vi "Set_Tunnel_Speed.vi"(3 "Mode":T1, 5 "Tunnel Velocity m/s":dbl min=0.0 max=50.0 format="%.2f") -> (0 "Error String":string)   [LabVIEW 2010]
doc: "This is an example of using features of the VI Server as a client. It shows how you might browse from one or more applications that may be exporting data from one or more data stations. \n\nThe example shows how to query a server for its list of exported VIs, how to get references to the VIs, and how call them with the Call By Reference function."
uses:
  Sub VIs/ADAM Controls/Tunnel_speed_mode.ctl
  Anemometry/Anemometry Sub Vis/File/Setup_Filetype.ctl
  Sub VIs/ADAM Controls/Channel_State.ctl
  Sub VIs/ADAM Controls/Calib_type_ADAM.ctl
  Sub VIs/ADAM Controls/Module_type_ADAM.ctl
  Sub VIs/ADAM Controls/Ch_description_ADAM.ctl
  Sub VIs/ADAM Controls/Function_ADAM.ctl
  Sub VIs/ADAM Controls/Address.ctl
  Anemometry/Anemometry Sub Vis/Controls/Global_mode.ctl
  Sub VIs/ADAM Controls/Update_scan_value.ctl
  Anemometry/Anemometry Sub Vis/Globals/Preference_global.vi
  Anemometry/Anemometry Sub Vis/Globals/Trav_pos_global.vi
  Anemometry/Anemometry Sub Vis/Globals/Constants_global.vi
  <vilib>/Analysis/NI_AALBase.lvlib
panel:
  in  "Set EnFlo Tun Speed":refnum<vi>
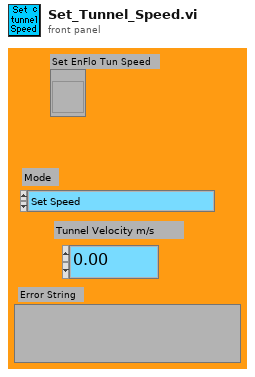
[diagram p1: front panel]
types:
  T1 = typedef "Tunnel_speed_mode.ctl" = enum16{"Set Speed", "Set Speed then wait", "Is tunnel speed allowable?"}
  T2 = typedef "Setup_Filetype.ctl" = enum16{"Measurement Setups", "Calibration Setups", "General", "Results File Plotter Setups", "Speed Calib Tweaks"}
  T3 = typedef "Channel_State.ctl" = enum16{"On", "Off", "Always On", "Always Off"}
  T4 = typedef "Calib_type_ADAM.ctl" = enum16{"Raw", "Bx + A", "Cx^2 + Bx + A", "Dx^3 + Cx^2 + Bx + A", "In Band", "Hi-Tec Q", "Hi-Tec M_dot", "Text"}
  T5 = typedef "Module_type_ADAM.ctl" = enum16{"4011", "4012", "4013", "4014", "4016", "4017", "4018", "4021", "4050", "4052", "4053", "4060", "4080", "5000", "5017", "5018", "5024", "5051", "5056", "5060", "6060", "Tracker", "WEST", "GILL", "JEM", "VICI", "Vaisala", "DRUCK", "Run VI Named:", "IR2100", "PPT", "Comparator", "VIRTUAL", "Hold Value", "Read A", "Read Ch", "Coded", "Client Info", "Web Client", "X10", "Test"}
  T6 = typedef "Ch_description_ADAM.ctl" = cluster{"Ch Name":string, "Type":T5, "Function":T7, "Ch State":T3, "Calibration type":T4, "A":dbl, "B":dbl, "C":dbl, "D":dbl, "Comments":string, "Address":T8, "String":string, "Duty":u16}
  T7 = typedef "Function_ADAM.ctl" = enum16{"Analogue Input", "Digital Input", "Event counter", "Event rate", "Analogue Output", "Digital Output", "Relay Output"}
  T8 = typedef "Address.ctl" = cluster{"Main":i32, "Ch.":i32, "Sub":i32, "Port Name":string}
  T9 = typedef "Global_mode.ctl" = enum16{"Read Global", "Load Global From File", "Write Global to File"}
  T10 = typedef "Update_scan_value.ctl" = cluster{"Channel Name":string, "New Value":dbl}
  T11 = typedef "Server_Comms.ctl" = enum16{"Server Link Healthy", "Do Not Link To Server"}
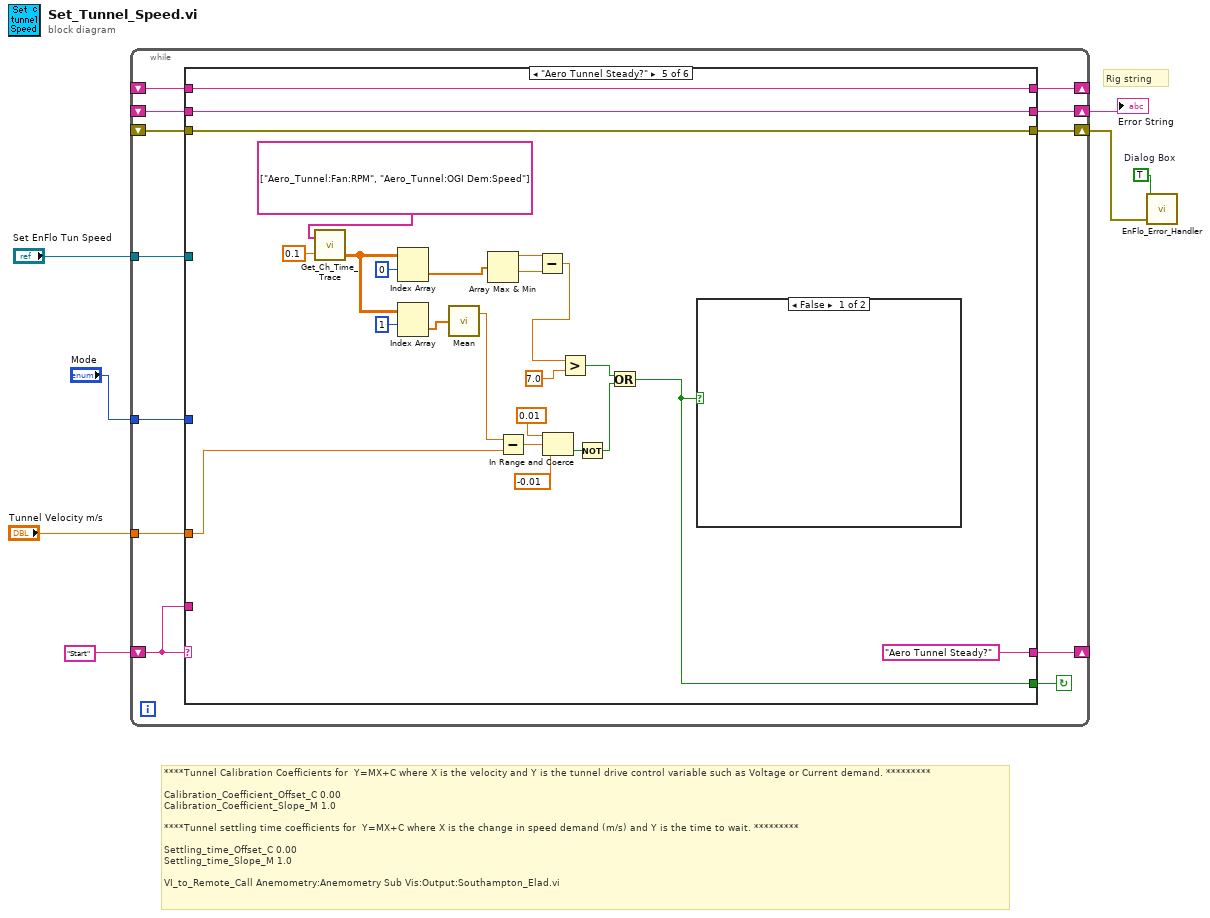
[diagram p0: block diagram]
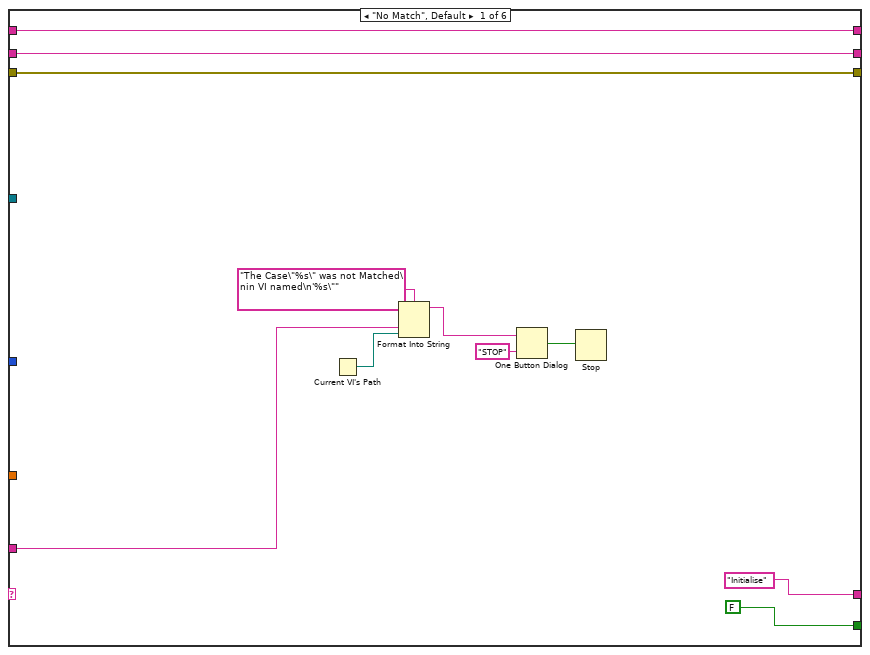
[diagram p2: hidden frame]
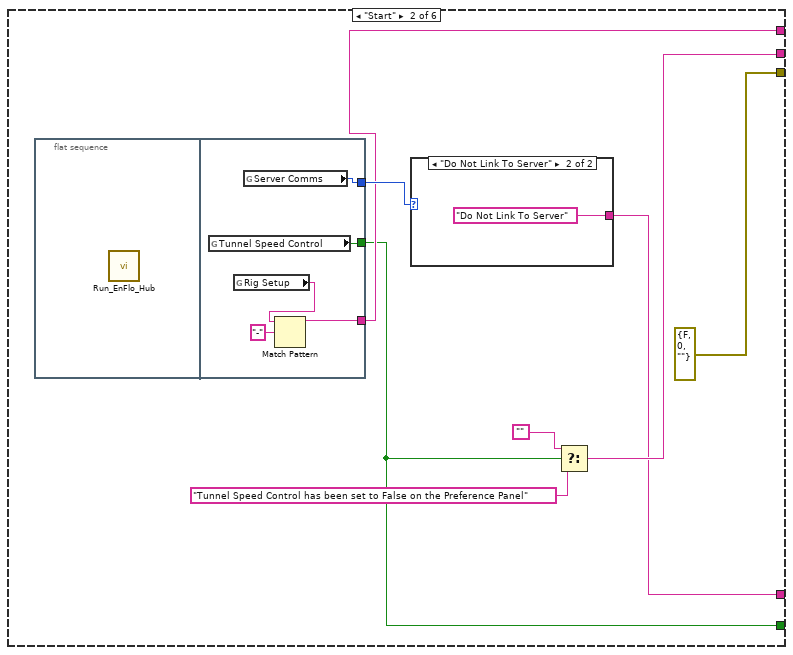
[diagram p3: hidden frame]
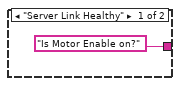
[diagram p4: hidden frame]
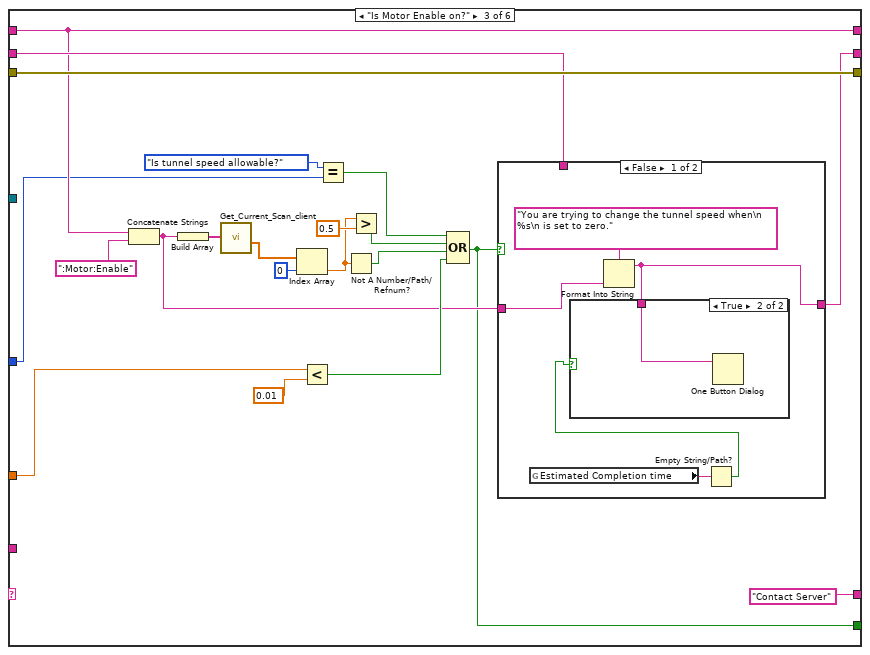
[diagram p5: hidden frame]
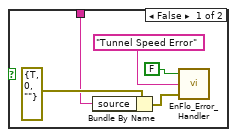
[diagram p6: hidden frame]
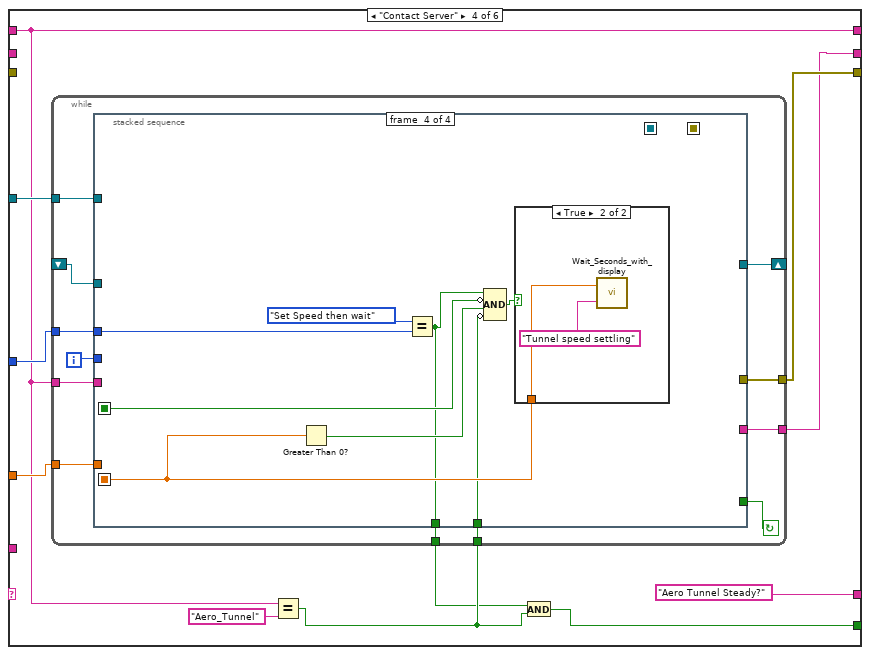
[diagram p8: hidden frame]
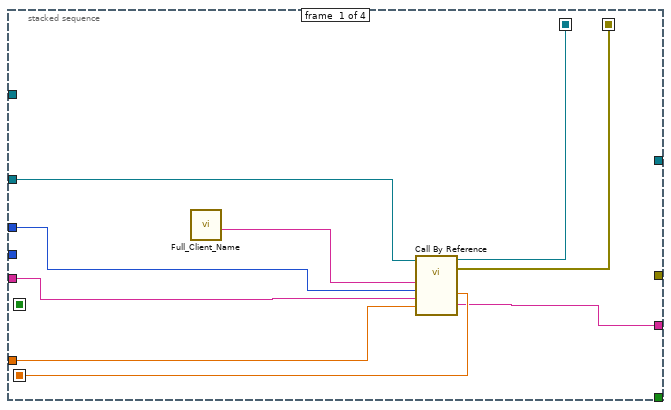
[diagram p9: hidden frame]
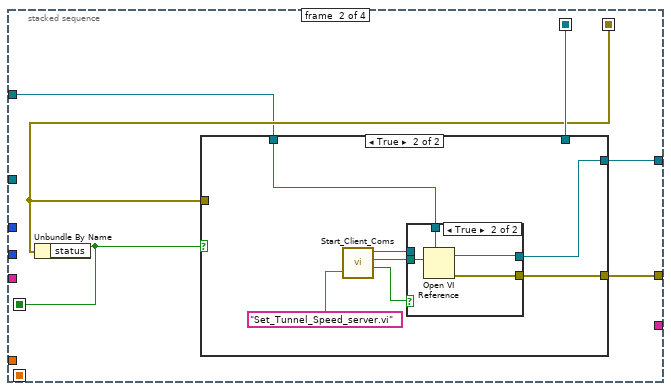
[diagram p10: hidden frame]
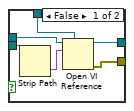
[diagram p12: hidden frame]
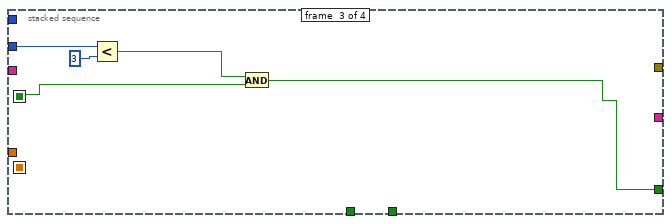
[diagram p13: hidden frame]
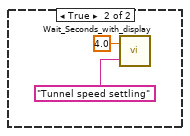
[diagram p15: hidden frame]
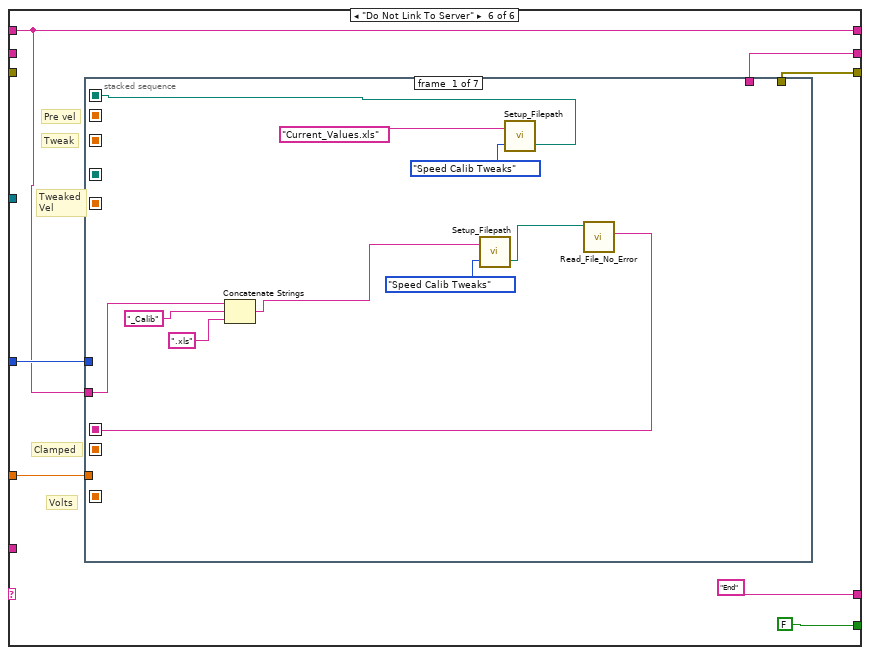
[diagram p16: hidden frame]
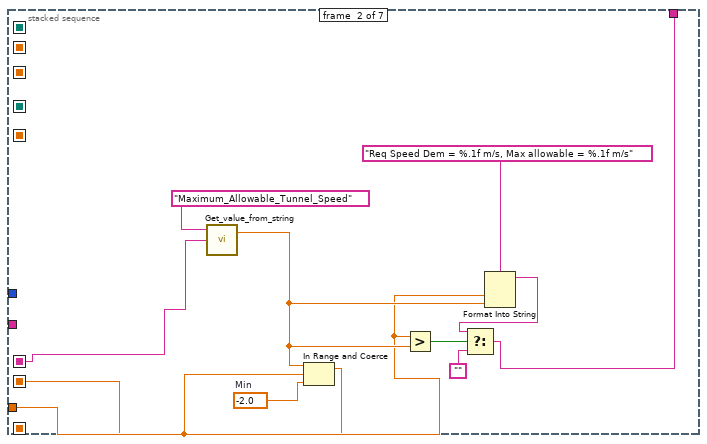
[diagram p17: hidden frame]
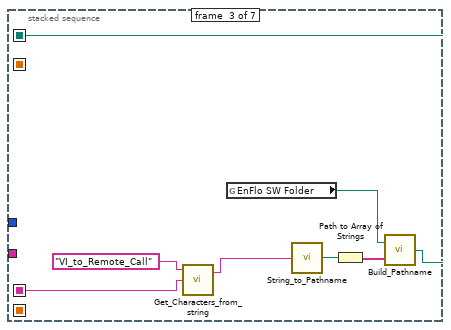
[diagram p18: hidden frame]
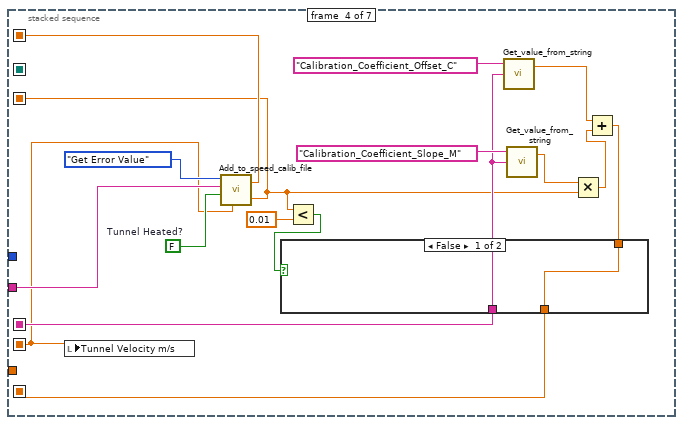
[diagram p19: hidden frame]
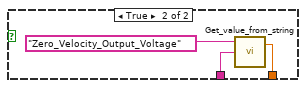
[diagram p20: hidden frame]
diagram:
  w7 = TRUE  # Dialog Box
  # "Rig string"
  # "****Tunnel Calibration Coefficients for  Y=MX+C where X is the velocity and Y is the tunnel drive control variable such as Voltage or Current demand. *********\n\nCalibration_Coefficient_Offset_C\t0.00\nCalibration_Coefficient_Slope_M\t1.0\n\n****Tunnel settling time coefficients for  Y=MX+C where X is the change in speed demand (m/s) and Y is the time to wait. *********\n\nSettling_time_Offset_C\t0.00\nSettling_time_Slope_M\t1.0\n\nVI_to_Remote_Call\tAnemometry:Anemometry Sub Vis:Output:Southampton_Elad.vi"
  n1 = while {
    shift-left: "Start" -> [w18]
    shift-right: [w19] -> _
    shift-right: [w17] -> w5
    shift-left: _ -> [w16]
    shift-right: [w15] -> w4
    shift-left: _ -> [w10]
    tunnel: "Mode" -> [w14]
    tunnel: "Tunnel Velocity m/s" -> [w13]
    shift-right: [w12] -> _
    shift-left: _ -> [w11]
    tunnel: "Set EnFlo Tun Speed" -> [w8]
    stop <- w9 continue-if-true
    n2 = case shown="\"Aero Tunnel Steady?\"" w18 {
      tunnel: [FALSE w35 w51 w79 w156 FALSE] -> w9
      tunnel: ["Initialise" w31 "Contact Server" ("f") "Aero Tunnel Steady?" ("f") "Aero Tunnel Steady?" ("f") "End"] -> w19
      tunnel: w18 -> [w25 _ _ _ _ _]
      tunnel: [w22 w33 w53 w86 w172 w179] -> w17
      tunnel: w16 -> [w22 _ w52 _ w172 _]
      tunnel: [w20 errorcluster {"status"=FALSE, "code"=0, "source"=""} ("error out") w55 w87 w171 w178] -> w15
      tunnel: w14 -> [_ _ w48 w89 _ w181]
      tunnel: w13 -> [_ _ w56 w88 w163 w180]
      tunnel: [w21 w36 w50 w83 w173 w177] -> w12
      tunnel: w11 -> [w21 _ w50 w83 w173 w177]
      tunnel: w10 -> [w20 _ w55 _ w171 _]
      tunnel: w8 -> [_ _ _ w85 _ _]
      frame "No Match", Default {
        n3 = Current VI's Path() -> (path=w24:path)
        n4 = Format Into String(format string="The Case\"%s\" was not Matched\nin VI named\n'%s\"" ("Format String"), w25, w24) -> (resulting string=w28:string)  [unwired: 2 in, 1 out]
        n5 = One Button Dialog(message=w28, button name ("OK")="STOP") -> (true=w26:bool)
        n6 = Stop(stop? (T)=w26) -> ()
      }
      frame "Start" {
        n7 = flat-sequence {
          tunnel: [w45] -> w38
          tunnel: [w44] -> w35
          tunnel: [w41] -> w36
          frame #0 {
            n8 = call "Run_EnFlo_Hub.vi"() -> ()  [unwired: 8 out]
          }
          frame #1 {
            n9 = global read "Preference_global.vi" "Tunnel Speed Control"() -> (w44:bool)
            n10 = global read "Preference_global.vi" "Rig Setup"() -> (w43:string)
            n11 = global read "Preference_global.vi" "Server Comms"() -> (w45:T11)
            n12 = Match Pattern(string=w43, regular expression="-") -> (before substring=w41:string)  [unwired: 4 out]
          }
        }
        n13 = case shown="\"Do Not Link To Server\"" w38 {
          tunnel: ["Is Motor Enable on?" "Do Not Link To Server"] -> w31
          frame "Server Link Healthy" {
          }
          frame "Do Not Link To Server" {
          }
        }
        n14 = Select(t="", s=w35, f="Tunnel Speed Control has been set to False on the Preference Panel" ("Error String")) -> (s? t:f=w33:string)
      }
      frame "Is Motor Enable on?" {
        n15 = Concatenate Strings(w50, ":Motor:Enable" ("string")) -> (w54:string)
        n16 = Build Array(w54) -> (w58:string[])
        n17 = call "Get_Current_Scan_client.vi"("ADAM Ch Names"=w58) -> ("Numerical Values"=w59:dbl[])  [unwired: 3 out]
        n18 = Index Array(array=w59, index=0) -> (element=w61:dbl)
        n19 = Less?(x=w56, y=0.01) -> (x < y?=w66:bool)
        n20 = Equal?(x=Tunnel_speed_mode."Is tunnel speed allowable?" ("Mode"), y=w48) -> (x = y?=w47:bool)
        n21 = Not A Number/Path/Refnum?(number/path/refnum=w61) -> (NaN/Path/Refnum?=w63:bool)
        n22 = Greater?(x=w61, y=0.5) -> (0:w64:bool)
        n23 = Compound Arithmetic op=OR(w47, w64, w63, w66) -> (w51:bool)
        n24 = case shown="False" w51 {
          tunnel: w54 -> [w70 _]
          tunnel: [w67 w78] -> w53
          tunnel: w52 -> [_ w78]
          frame False {
            n25 = global read "Trav_pos_global.vi" "Estimated Completion time"() -> (w69:string)
            n26 = Format Into String(format string="You are trying to change the tunnel speed when\n %s\n is set to zero.", w70) -> (resulting string=w67:string)  [unwired: 2 in, 1 out]
            n27 = Empty String/Path?(string/path=w69) -> (empty?=w68:bool)
            n28 = case shown="True" w68 {
              tunnel: w67 -> [w73 w77]
              frame False {
                n29 = Bundle By Name(cluster=errorcluster {"status"=TRUE, "code"=0, "source"=""} ("error in (no error)"), "source"=w73) -> (w74:errorcluster)
                n30 = call "EnFlo_Error_Handler.vi"("error in (no error)"=w74, "Error Type"="Tunnel Speed Error", "Dialog Box (T)"=FALSE) -> ()  [unwired: 3 out]
              }
              frame True {
                n31 = One Button Dialog(message=w77) -> ()  [unwired: 2 out]
              }
            }
          }
          frame True {
          }
        }
      }
      frame "Contact Server" {
        n32 = Equal?(x=w83, y="Aero_Tunnel") -> (x = y?=w81:bool)
        n33 = while {
          tunnel: w89 -> [w96]
          tunnel: w88 -> [w97]
          tunnel: [w98] -> w87
          shift-left: _ -> [w93]
          shift-right: [w101] -> _
          tunnel: [w95] -> w86
          tunnel: w83 -> [w94]
          tunnel: w85 -> [w92]
          tunnel: w81 -> [w91]
          tunnel: [w90] -> w80
          i -> [w100]
          stop <- w99 continue-if-true
          n34 = stacked-sequence {
            seq-local: [w109 _ _ _] -> [_ w115 _ _]
            seq-local: [w108 _ _ _] -> [_ w113 _ _]
            seq-local: [_ w114 _ _] -> [_ _ w137 w144]
            seq-local: [w105 _ _ _] -> [_ _ _ w147]
            tunnel: w93 -> [w110 _ _ _]
            tunnel: [_ w116 _ _] -> w101
            tunnel: w100 -> [_ _ w138 _]
            tunnel: [_ _ w136 _] -> w99
            tunnel: [_ w112 _ _] -> w98
            tunnel: w97 -> [w106 _ _ _]
            tunnel: w96 -> [w102 _ _ w148]
            tunnel: [w104 _ _ _] -> w95
            tunnel: w94 -> [w103 _ _ _]
            tunnel: w92 -> [_ w111 _ _]
            tunnel: w91 -> [_ _ _ w142]
            tunnel: [_ _ _ w141] -> w90
            frame #0 {
              n35 = call "Full_Client_Name.vi"() -> ("Client Name"=w107:string)
              n36 = call-by-ref "?"(reference=w110, "Tunnel Velocity m/s"=w106, "Rig Name"=w103, "Mode"=w102, "Client Name"=w107) -> (reference out=w109:refnum<vi>, error out=w108:errorcluster, "Error String"=w104:string, "Settling Time (s)"=w105:dbl)  [unwired: 1 in, 1 out]
            }
            frame #1 {
              n37 = Unbundle By Name(w113) -> ("status"=w114:bool)
              n38 = case shown="True" w114 {
                tunnel: [w117 w121] -> w116
                tunnel: w115 -> [w117 _]
                tunnel: [w118 w120] -> w112
                tunnel: w113 -> [w118 _]
                tunnel: w111 -> [_ w119]
                frame False {
                }
                frame True {
                  n39 = call "Start_Client_Coms.vi"("VI name to run on server"="Set_Tunnel_Speed_server.vi") -> ("LabVIEW application reference"=w123:refnum<vi>, "Checked VI name"=w124:path, "Local Call"=w122:bool)  [unwired: 1 in, 1 out]
                  n40 = case shown="True" w122 {
                    tunnel: [w130 w135] -> w121
                    tunnel: w119 -> [w128 w134]
                    tunnel: w124 -> [w127 w133]
                    tunnel: w123 -> [w126 _]
                    tunnel: [w129 w132] -> w120
                    frame False {
                      n41 = Strip Path(path=w127) -> (name=w131:string)  [unwired: 1 out]
                      n42 = Open VI Reference(type specifier VI Refnum (for type only)=w128, application reference (local)=w126, vi path=w131) -> (vi reference=w130:refnum<vi>, error out=w129:errorcluster)  [unwired: 1 in, 2 out]
                    }
                    frame True {
                      n43 = Open VI Reference(type specifier VI Refnum (for type only)=w134, vi path=w133) -> (vi reference=w135:refnum<vi>, error out=w132:errorcluster)  [unwired: 1 in, 3 out]
                    }
                  }
                }
              }
            }
            frame #2 {
              n44 = Less?(x=w138, y=3) -> (x < y?=w140:bool)
              n45 = And(x=w140, y=w137) -> (x .and. y?=w136:bool)
            }
            frame #3 {
              n46 = Greater Than 0?(x=w147) -> (x > 0?=w143:bool)
              n47 = Equal?(x=Tunnel_speed_mode."Set Speed then wait" ("Mode"), y=w148) -> (x = y?=w141:bool)
              n48 = Compound Arithmetic op=AND(w141, invert w144, w143, invert w142) -> (w145:bool)
              n49 = case shown="True" w145 {
                tunnel: w147 -> [_ w149]
                frame False {
                }
                frame True {
                  n50 = call "Wait_Seconds_with_display.vi"("Message"="Tunnel speed settling", "Seconds to wait"=w149) -> ()  [unwired: 2 out]
                }
              }
            }
          }
        }
        n51 = And(x=w80, y=w81) -> (x .and. y?=w79:bool)
      }
      frame "Aero Tunnel Steady?" {
        n52 = call "Get_Ch_Time_Trace.vi"("Desired Ch Names"=string[] ["Aero_Tunnel:Fan:RPM", "Aero_Tunnel:OGI Dem:Speed"] ("ADAM Ch Names"), "History Length (mins)"=0.1) -> ("Output array"=w166:dbl[][])  [unwired: 2 out]
        n53 = Index Array(array=w166, index (row)=0) -> (element=w162:dbl[])  [unwired: 1 in]
        n54 = Index Array(array=w166, index (row)=1) -> (element=w165:dbl[])  [unwired: 1 in]
        n55 = call <vilib>:"Mean.vi"("X"=w165) -> ("mean"=w164:dbl)  [unwired: 1 out]
        n56 = Array Max & Min(array=w162) -> (max value=w161:dbl, min value=w160:dbl)  [unwired: 2 out]
        n57 = Subtract(x=w164, y=w163) -> (x-y=w153:dbl)
        n58 = Subtract(x=w161, y=w160) -> (x-y=w159:dbl)
        n59 = In Range and Coerce(upper limit=0.01, x=w153, lower limit=-0.01) -> (In Range?=w152:bool)  [unwired: 1 out]
        n60 = Greater?(x=w159, y=7.0) -> (0:w157:bool)
        n61 = Not(x=w152) -> (.not. x?=w151:bool)
        n62 = Or(x=w157, y=w151) -> (x .or. y?=w156:bool)
        n63 = case shown="False" w156 {
          frame False {
          }
          frame True {
            n64 = call "Wait_Seconds_with_display.vi"("Message"="Tunnel speed settling", "Seconds to wait"=4.0) -> ()  [unwired: 2 out]
          }
        }
      }
      frame "Do Not Link To Server" {
        # "Clamped"
        # "Pre vel"
        # "Tweak"
        # "Tweaked\nVel"
        # "Volts"
        n65 = stacked-sequence {
          seq-local: [w190 _ _ _ _ _ _] -> [_ w204 w210 w218 w234 w293 _]
          seq-local: [_ _ w205 _ _ _ _] -> [_ _ _ _ w238 _ _]
          seq-local: [_ _ _ w214 _ _ _] -> [_ _ _ _ w233 _ w306]
          seq-local: [_ _ _ w217 _ _ _] -> [_ _ _ _ w236 w288 _]
          seq-local: [_ _ _ _ w235 _ _] -> [_ _ _ _ _ w287 _]
          seq-local: [_ _ _ w219 _ _ _] -> [_ _ _ _ _ _ w312]
          seq-local: [w187 _ _ _ _ _ _] -> [_ _ _ _ _ _ w314]
          seq-local: [_ w195 _ _ _ _ _] -> [_ _ _ w212 _ _ w311]
          tunnel: w180 -> [_ w196 _ _ _ _ _]
          tunnel: w177 -> [w191 _ _ w227 _ _ w308]
          tunnel: w181 -> [_ _ _ _ w237 w282 _]
          tunnel: [_ w194 _ _ _ _ _] -> w179
          tunnel: [_ _ _ _ w232 _ _] -> w178
          frame #0 {
            n66 = Concatenate Strings(w191, "_Calib" ("Substring"), ".xls" ("string")) -> (w185:string)
            n67 = call "Setup_Filepath.vi"("Setup File Type"=Setup_Filetype."Speed Calib Tweaks", "Filename in"=w185) -> ("Filename Out"=w184:path)  [unwired: 1 out]
            n68 = call "Setup_Filepath.vi"("Setup File Type"=Setup_Filetype."Speed Calib Tweaks", "Filename in"="Current_Values.xls" ("name or relative path")) -> ("Filename Out"=w187:path)  [unwired: 1 out]
            n69 = call "Read_File_No_Error.vi"("Filename"=w184) -> ("string"=w190:string)  [unwired: 2 in, 7 out]
          }
          frame #1 {
            w198 = -2.0  # Min
            n70 = call "Get_value_from_string.vi"("Input string"=w204, "Variable name"="Maximum_Allowable_Tunnel_Speed") -> ("Value"=w197:dbl)  [unwired: 1 in, 1 out]
            n71 = In Range and Coerce(upper limit=w197, x=w196, lower limit=w198) -> (coerced(x)=w195:dbl)  [unwired: 1 out]
            n72 = Greater?(x=w196, y=w197) -> (0:w199:bool)
            n73 = Format Into String(format string="Req Speed Dem = %.1f m/s, Max allowable = %.1f m/s", w196, w197) -> (resulting string=w201:string)  [unwired: 2 in, 1 out]
            n74 = Select(t=w201, s=w199, f="") -> (s? t:f=w194:string)
          }
          frame #2 {
            n75 = call "Get_Characters_from_string.vi"("Input string"=w210, "Variable name"="VI_to_Remote_Call") -> ("Value"=w208:string)  [unwired: 1 in, 1 out]
            n76 = global read "Constants_global.vi" "EnFlo SW Folder"() -> (w206:path)
            n77 = call "String_to_Pathname.vi"("Input String"=w208) -> ("path"=w209:path)
            n78 = Path to Array of Strings(0:w209) -> (2:w207:string[])  [unwired: 1 out]
            n79 = call "Build_Pathname.vi"("Output Array"=w207, "Pathname"=w206) -> ("Appended path"=w205:path)
          }
          frame #3 {
            w225 = FALSE  # Tunnel Heated?
            n80 = local write "Tunnel Velocity m/s"(w212) -> ()
            n81 = call "Add_to_speed_calib_file.vi"("Desired Velocity"=w212, "Tunnel Heated?"=w225, "Rig Name"=w227, "Mode"=enum16{"Add Row", "Get Error Value"}."Get Error Value") -> ("Tweaked Demand"=w217:dbl, "Calib Tweak %"=w219:dbl)  [unwired: 2 in]
            n82 = Less?(x=w217, y=0.01) -> (x < y?=w215:bool)
            n83 = call "Get_value_from_string.vi"("Input string"=w218, "Variable name"="Calibration_Coefficient_Offset_C") -> ("Value"=w220:dbl)  [unwired: 1 in, 1 out]
            n84 = call "Get_value_from_string.vi"("Input string"=w218, "Variable name"="Calibration_Coefficient_Slope_M") -> ("Value"=w222:dbl)  [unwired: 1 in, 1 out]
            n85 = Multiply(x=w222, y=w217) -> (x*y=w221:dbl)
            n86 = Add(x=w220, y=w221) -> (x+y=w213:dbl)
            n87 = case shown="False" w215 {
              tunnel: w218 -> [_ w230]
              tunnel: [w228 w229] -> w214
              tunnel: w213 -> [w228 _]
              frame False {
              }
              frame True {
                n88 = call "Get_value_from_string.vi"("Input string"=w230, "Variable name"="Zero_Velocity_Output_Voltage") -> ("Value"=w229:dbl)  [unwired: 1 in, 1 out]
              }
            }
          }
          frame #4 {
            n89 = while {
              tunnel: w238 -> [w248]
              tunnel: w237 -> [w247]
              tunnel: w236 -> [w246]
              tunnel: [w245] -> w235
              shift-right: [w243] -> _
              shift-left: _ -> [w242]
              tunnel: [w241] -> w232
              tunnel: w234 -> [w240]
              tunnel: w233 -> [w239]
              stop <- TRUE stop-if-true
              n90 = case shown="\"Set Speed then wait\", Default" w247 {
                tunnel: w248 -> [_ w268]
                tunnel: w246 -> [_ w255]
                tunnel: [w250 w257] -> w245
                tunnel: [w250 w255] -> w243
                tunnel: w242 -> [w250 w256]
                tunnel: [errorcluster {"status"=FALSE, "code"=0, "source"=""} ("error out") w251] -> w241
                tunnel: w240 -> [_ _]
                tunnel: w239 -> [_ w254]
                frame "Is tunnel speed allowable?" {
                }
                frame "Set Speed then wait", Default {
                  n91 = Open VI Reference(type specifier VI Refnum (for type only)=refnum<vi> refnum, vi path=w268) -> (vi reference=w266:refnum<vi>, error out=w265:errorcluster)  [unwired: 1 in, 3 out]
                  n92 = property class="VI Interface Type 0"(reference=w266, error in=w265) -> (reference out=w263:refnum<vi>, error out=w264:errorcluster, "Front Panel.Open"=w262:bool)
                  n93 = case shown="False" w262 {
                    tunnel: w264 -> [w273 w276]
                    tunnel: w263 -> [w272 w277]
                    tunnel: [w271 w277] -> w261
                    tunnel: [w270 w276] -> w260
                    tunnel: [0.0 ("Tweaked Demand") w275] -> w257
                    tunnel: w256 -> [_ w275]
                    frame False {
                      n94 = property class="VI Interface Type 0"(reference=w272, error in=w273, "Front Panel.Open"=TRUE ("Front Panel Window:Open")) -> (reference out=w271:refnum<vi>, error out=w270:errorcluster)
                    }
                    frame True {
                    }
                  }
                  n95 = call-by-ref "?"(reference=w261, error in=w260, "Demand"=w254) -> (reference out=w258:refnum<vi>, error out=w259:errorcluster, "error out"=w252:errorcluster)
                  n96 = Close Reference(reference=w258, error in (no error)=w259) -> (error out=w253:errorcluster)
                  n97 = Select(t=w253, s=w253, f=w252) -> (s? t:f=w251:errorcluster)
                }
              }
            }
          }
          frame #5 {
            n98 = Subtract(x=w287, y=w288) -> (x-y=w286:dbl)
            n99 = Absolute Value(x=w286) -> (abs(x)=w280:dbl)
            n100 = call "Get_value_from_string.vi"("Input string"=w293, "Variable name"="Settling_time_Offset_C") -> ("Value"=w289:dbl)  [unwired: 1 in, 1 out]
            n101 = call "Get_value_from_string.vi"("Input string"=w293, "Variable name"="Settling_time_Slope_M") -> ("Value"=w291:dbl)  [unwired: 1 in, 1 out]
            n102 = Multiply(x=w291, y=w280) -> (x*y=w290:dbl)
            n103 = Add(x=w289, y=w290) -> (x+y=w281:dbl)
            n104 = Greater?(x=w280, y=0.05) -> (0:w278:bool)
            n105 = Equal?(x=Tunnel_speed_mode."Set Speed then wait" ("Mode"), y=w282) -> (x = y?=w284:bool)
            n106 = Compound Arithmetic op=AND(w278, w284) -> (w283:bool)
            n107 = case shown="False" w283 {
              tunnel: w281 -> [_ w295]
              frame False {
              }
              frame True {
                n108 = call "Wait_Seconds_with_display.vi"("Message"="Tunnel speed settling", "Seconds to wait"=w295) -> ()  [unwired: 2 out]
              }
            }
          }
          frame #6 {
            n109 = Concatenate Strings(w308, ":Speed:Dem_Voltage" ("string")) -> (w303:string)
            n110 = Bundle By Name(cluster=T10 {"Channel Name"="", "New Value"=0.0} ("Update Scan Value Cluster"), "Channel Name"=w303, "New Value"=w306) -> (w309:T10)
            n111 = call "Value_to_string.vi"("Value"=w312, "Label for value"="Calib Tweak") -> ("Output string"=w317:string)  [unwired: 1 in]
            n112 = call "Value_to_string.vi"("Value"=w311, "Label for value"="Velocity Demand") -> ("Output string"=w316:string)  [unwired: 1 in]
            n113 = Concatenate Strings(w317, w316) -> (w315:string)
            n114 = Bundle By Name(cluster=T6 {"Ch Name"="", "Type"=enum."4011", "Function"=enum."Analogue Input", "Ch State"=enum."On", "Calibration type"=enum."Raw", "A"=0.0, "B"=0.0, "C"=0.0, "D"=0.0, "Comments"="", "Address"={"Main"=0, "Ch."=0, "Sub"=0, "Port Name"=""}, "String"="", "Duty"=0} ("Ch Discription"), "Ch Name"=w303, "Type"=Module_type_ADAM."Hold Value", "Calibration type"=Calib_type_ADAM."Raw", "Ch State"=Channel_State."On") -> (w297:T6)
            n115 = call "Write_File_Simple.vi"("append to file? (new file:F)"=FALSE, "character string"=w315, "file path"=w314) -> ()  [unwired: 2 out]
            n116 = Build Array(w309) -> (w299:T10[])
            n117 = Build Array(w297) -> (w298:T6[])
            n118 = call "Read_Write_Local_table.vi"("Mode"=Global_mode."Write Global to File", "Ch Values in"=w299, "Channels Descriptions In"=w298) -> ()  [unwired: 3 out]
          }
        }
      }
    }
  }
  "Error String" <- w5
  n119 = call "EnFlo_Error_Handler.vi"("error in (no error)"=w4, "Dialog Box (T)"=w7) -> ()  [unwired: 1 in, 3 out]
